vi "Pump Concentrations in ppm.vi"(11 "Pump Concetration in":T1 caption="Set Values Cluster") -> (3 "Pump Concentration out":T1 caption="Set Values Cluster")   [LabVIEW 2020, in "Linearisierung v2.lvlib" / "Gasteiler.lvlib" / "HovaCAL_Interface.lvlib" / "Helper.lvlib"]
uses:
  Helper.lvlib
  Controls/Pump Concentration.ctl
  Controls/Controls.lvlib
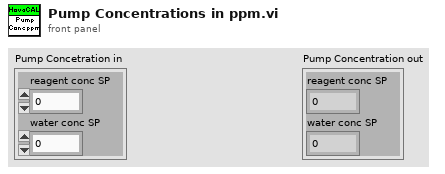
[diagram p1: front panel]
types:
  T1 = typedef "Linearisierung v2.lvlib/Gasteiler.lvlib/HovaCAL_Interface.lvlib/Controls.lvlib/Pump Concentration.ctl" = cluster{"reagent conc SP":dbl, "water conc SP":dbl}
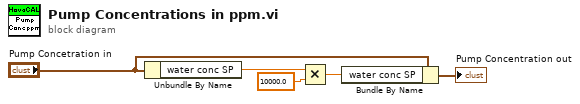
[diagram p0: block diagram]
diagram:
  n1 = Unbundle By Name("Pump Concetration in") -> ("water conc SP"=w3:dbl)
  n2 = Multiply(x=w3, y=10000.0) -> (x*y=w4:dbl)
  n3 = Bundle By Name(cluster="Pump Concetration in", "water conc SP"=w4) -> (→"Pump Concentration out":T1)
